vi "Assignment_Smart_Farming.vi"() -> ()   [LabVIEW 2020]
uses:
  <vilib>/MakerHub/LINX/Public/Peripherals/Digital/Digital Read 1 Chan.vi
  <vilib>/MakerHub/LINX/Public/Peripherals/Analog/Analog Read 1 Chan.vi
  <vilib>/MakerHub/LINX/Public/Peripherals/Digital/Digital Read N Chans.vi
  <vilib>/MakerHub/LINX/Public/Peripherals/Analog/Analog Read N Chans.vi
  <vilib>/MakerHub/LINX/Private/Local IO/LinxDigitalRead.vi
  <vilib>/MakerHub/LINX/Public/Utilities/Check Channel.vi
  <vilib>/MakerHub/LINX/Private/Local IO/LinxAnalogRead.vi
  <vilib>/MakerHub/LINX/Public/Utilities/Open Serial.vi
  <vilib>/MakerHub/LINX/Private/Utilties/Generate Error.vi
  <vilib>/httpClient/PUTBuffer.vi
  <vilib>/MakerHub/LINX/Public/Sensors/Motion/Servo/Servo Set Pulse Width One Channel.vi
  <vilib>/MakerHub/LINX/Public/Sensors/Motion/Servo/Servo Close One Channel.vi
  <vilib>/MakerHub/LINX/Public/Sensors/Motion/Servo/Servo Open One Channel.vi
  <vilib>/httpClient/LabVIEWHTTPClient.lvlib
  <vilib>/MakerHub/LINX/LMH-LINX.lvlib
  <vilib>/MakerHub/LINX/Public/Sensors/Motion/Servo/Servo.lvlib
panel:
  out "body":string
  out "PIR":bool
  out "Irrigation Level Received":dbl(slide) scale=0.0..10.0
  out "Rain Sensor":dbl(knob) scale=0.0..10.0
  out "Soil Moisture":dbl(slide) scale=0.0..50.0
  in  "STOP":bool
  out "Temp ^C":u8(knob) scale=0.0..50.0
  out "Humidity %":u8(knob) scale=0.0..100.0
  out "Device Name":string
  out "Data Sent":string
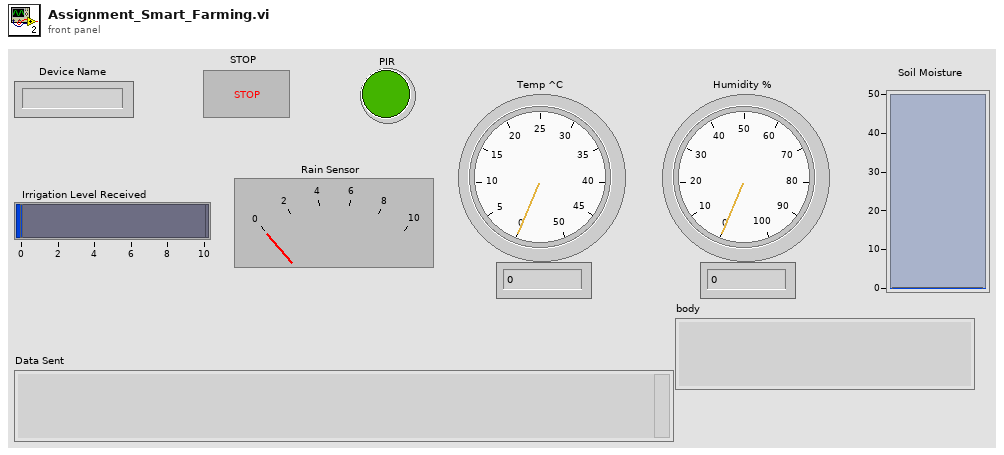
[diagram p1: front panel]
types:
  T1 = typedef "LMH-LINX.lvlib/LINX Ref.ctl" = cluster{"IO":T2, "Interface":T3, "LINX Device Config":T4}
  T2 = typedef "LMH-LINX.lvlib/Platform.ctl" = enum16{"Remote", "Local"}
  T3 = typedef "LMH-LINX.lvlib/Interface.ctl" = enum16{"Serial", "TCP"}
  T4 = typedef "LMH-LINX.lvlib/Device.lvlib/LINX Device Config.ctl" = cluster{"Interface":T3, "COM Port":refnum<visa-resource-name>, "TCP Configuration":T5, "Device Family":u8, "Device ID":u8, "Device Name":string, "TCP Ref":refnum<k5>, "Channels":T6}
  T5 = typedef "LMH-LINX.lvlib/Device.lvlib/TCP Config.ctl" = cluster{"IP Address":string, "Port":u16}
  T6 = typedef "LMH-LINX.lvlib/Channels.ctl" = cluster{"DI":u8[], "DO":u8[], "AI":u8[], "AO":u8[], "PWM":u8[], "QE":u8[], "UART":u8[], "I2C 2":u8[], "SPI":u8[], "CAN":u8[], "Servo":u8[], "AI Ref (V)":dbl, "AI Resolution (Bits)":u8, "AO Ref (V)":dbl, "AO Resolution (Bits)":u8}
  T7 = cluster{"Soil Moisture":dbl, "Rain":dbl, "Irrigation":string, "Humidity":i32, "Temperature":dbl, "PIR":bool}
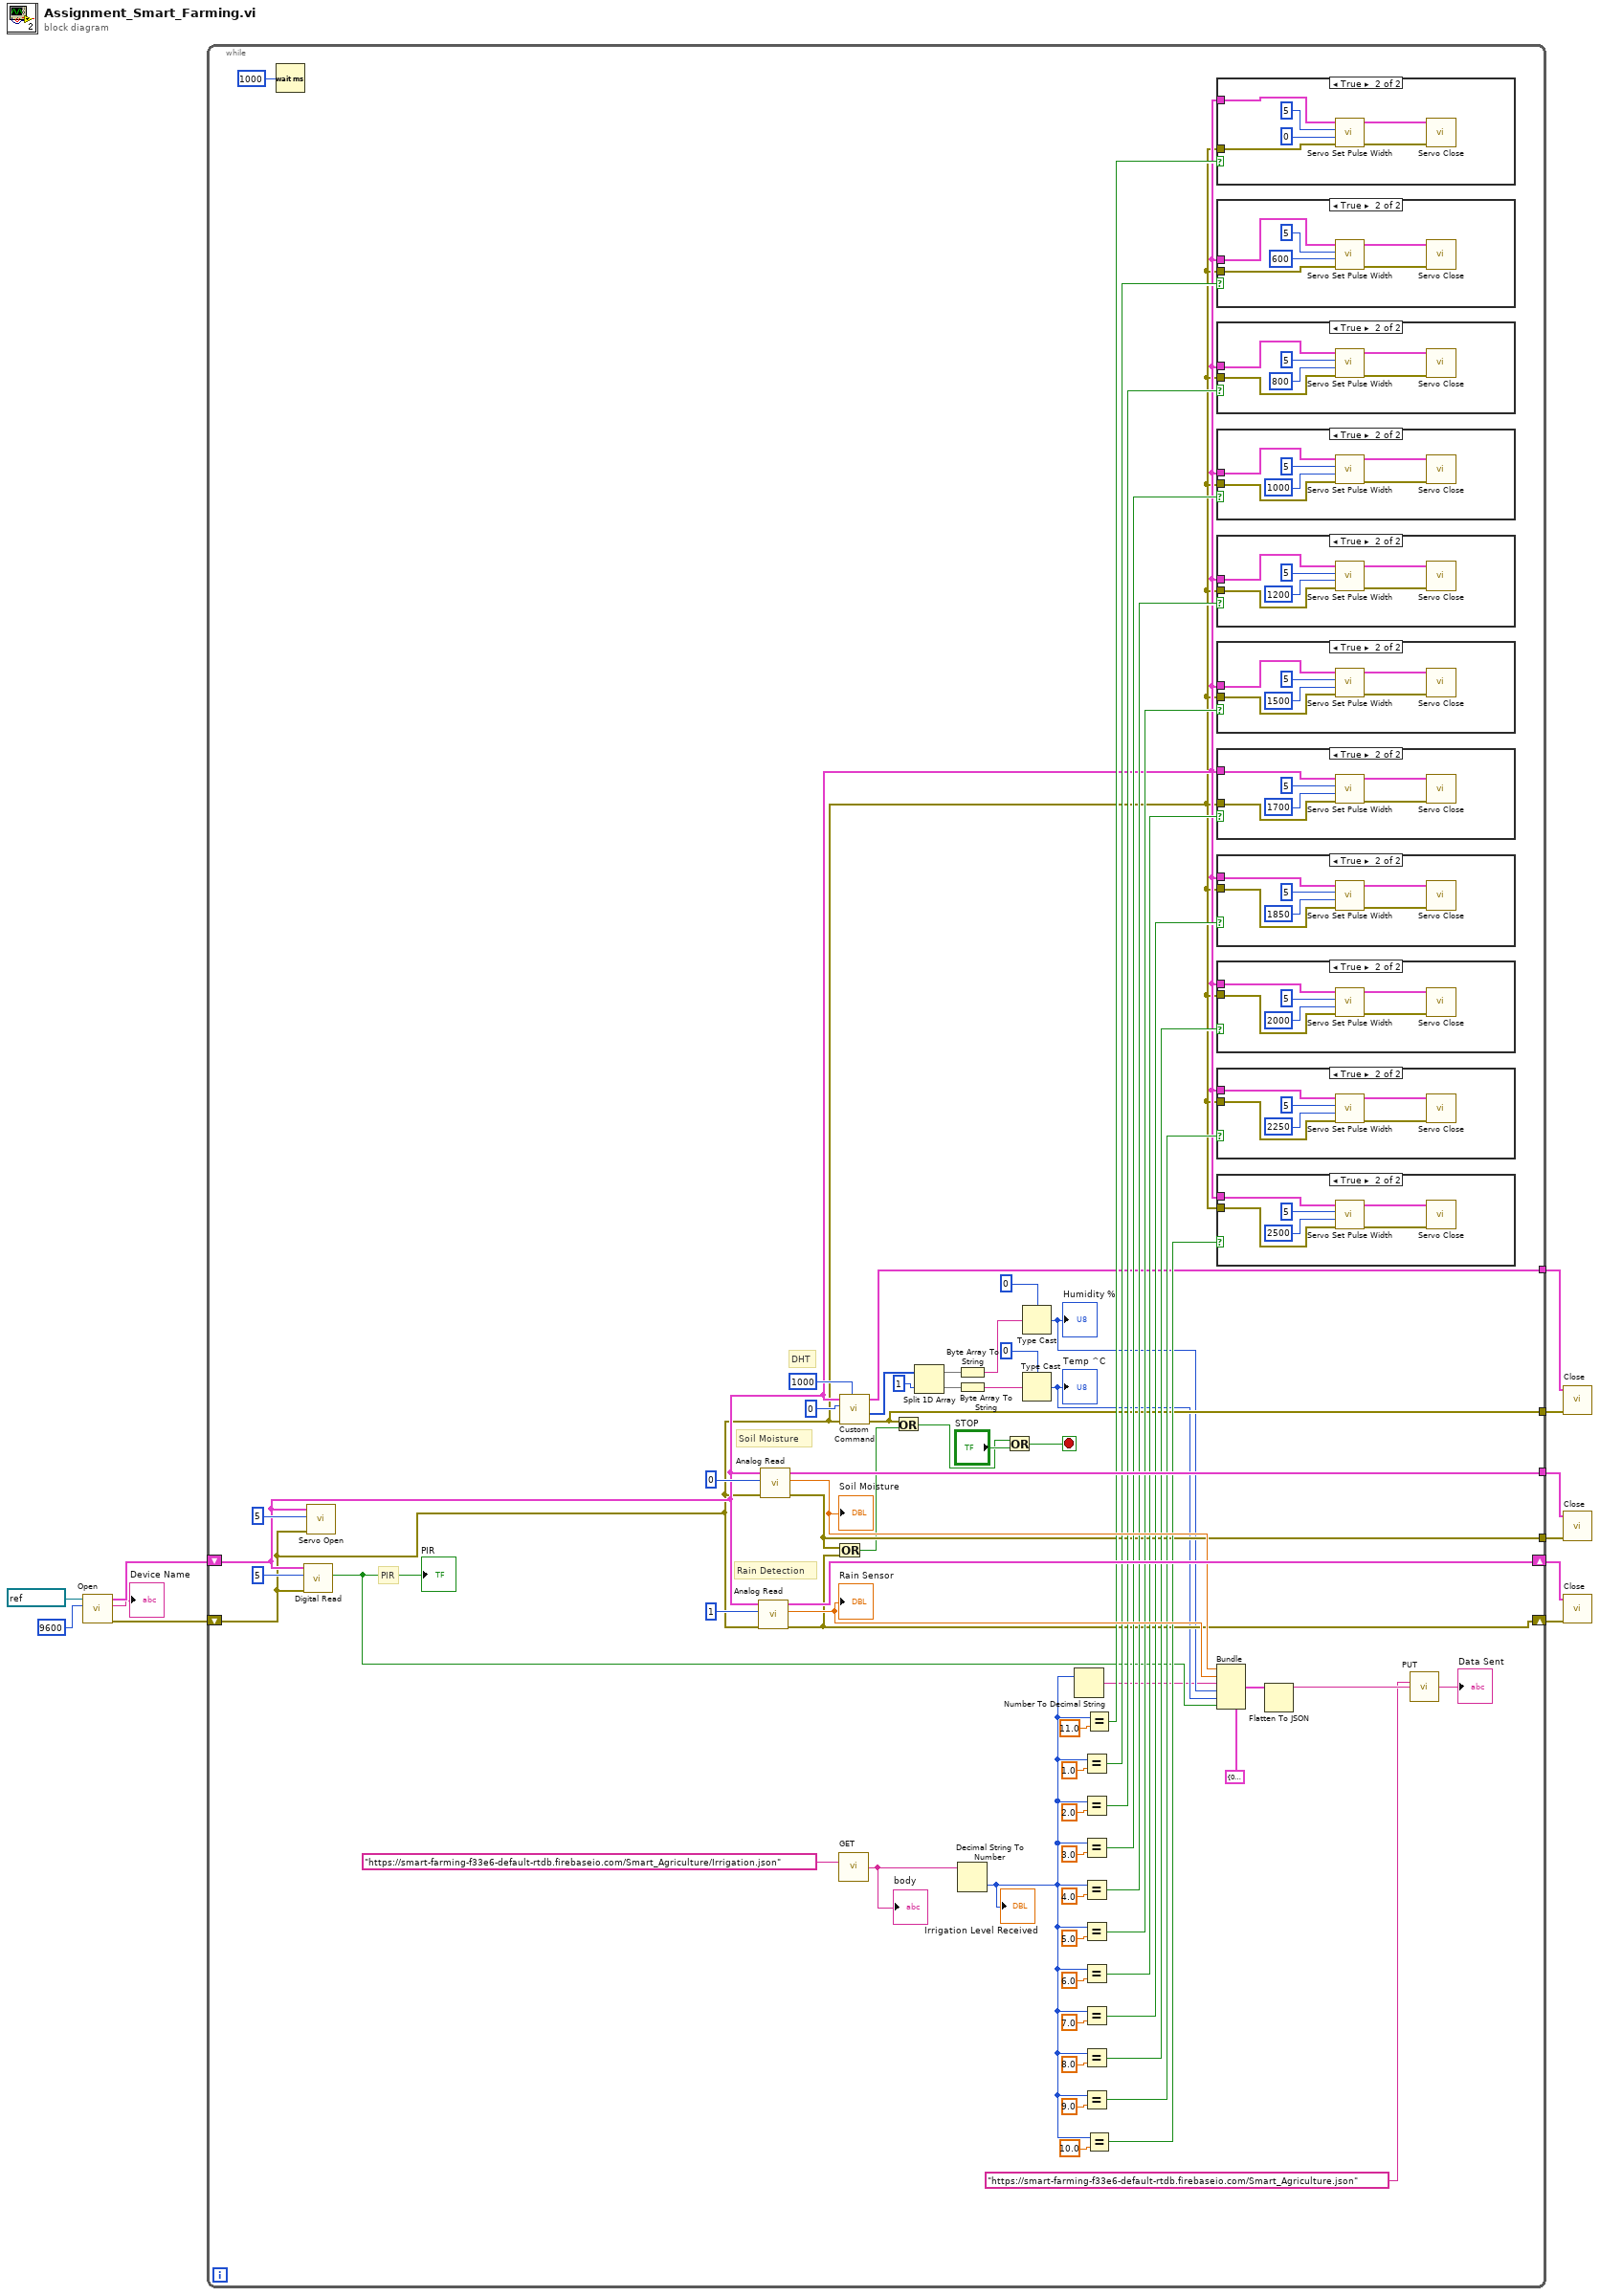
[diagram p0: block diagram]
diagram:
  n1 = call-poly <vilib>:"Open.vi"("Baud Rate Override"=u32 9600, "Serial Port"=refnum<visa-resource-name> "COM7") -> ("Error Out"=w8:errorcluster, "Device Name"=→"Device Name":string, "LINX Resource"=w9:T1)  [unwired: 7 in]
  n2 = while {
    tunnel: [w69] -> w5
    tunnel: [w28] -> w4
    shift-right: [w70] -> w7
    shift-left: w9 -> [w38]
    shift-right: [w27] -> w6
    shift-left: w8 -> [w37]
    tunnel: [w36] -> w2
    tunnel: [w26] -> w1
    stop <- w22 stop-if-true
    # "DHT"
    # "PIR"
    # "Rain Detection"
    # "Soil Moisture"
    n3 = Wait (ms)(milliseconds to wait=u32 1000) -> ()  [unwired: 1 out]
    n4 = call-poly <vilib>:"Digital Read.vi"("Error In"=w37, "DI Channel"=u8 5, "LINX Resource"=w38) -> ("DI Value"=w17:bool)  [unwired: 6 in, 2 out]
    "PIR" <- w17
    n5 = call-poly <vilib>:"Servo Open.vi"("Error In"=w37, "Servo Channel"=u8 5, "LINX Resource"=w38) -> ()  [unwired: 7 in, 2 out]
    n6 = call-poly <vilib>:"Analog Read.vi"("Error In"=w37, "Analog Channel"=u8 1, "LINX Resource"=w38) -> ("Error Out"=w27:errorcluster, "Voltage"=w64:dbl, "LINX Resource"=w70:T1)  [unwired: 5 in, 1 out]
    "Rain Sensor" <- w64
    n7 = call-poly <vilib>:"Analog Read.vi"("Error In"=w37, "Analog Channel"=u8 0, "LINX Resource"=w38) -> ("Error Out"=w28:errorcluster, "Voltage"=w65:dbl, "LINX Resource"=w69:T1)  [unwired: 5 in, 1 out]
    "Soil Moisture" <- w65
    n8 = Or(x=w28, y=w27) -> (x .or. y?=w25:bool)
    n9 = call <vilib>:"GET.vi"("url"="https://smart-farming-f33e6-default-rtdb.firebaseio.com/Smart_Agriculture/Irrigation.json") -> ("body"=w14:string)  [unwired: 11 in, 3 out]
    "body" <- w14
    n10 = call <vilib>:"Custom Command.vi"("Timeout (100 ms)"=1000, "Error In"=w37, "Custom Command Number"=u16 0, "LINX Resource"=w38) -> ("Error Out"=w26:errorcluster, "Response"=w20:u8[], "LINX Resource"=w36:T1)  [unwired: 4 in, 1 out]
    n11 = Or(x=w26, y=w25) -> (x .or. y?=w23:bool)
    n12 = Split 1D Array(array=w20, index=1) -> (first subarray=w34:u8[], second subarray=w33:u8[])
    n13 = Byte Array To String(unsigned byte array=w34) -> (string=w31:string)
    n14 = Byte Array To String(unsigned byte array=w33) -> (string=w29:string)
    n15 = Decimal String To Number(string=w14) -> (number=w13:i32)  [unwired: 2 in, 1 out]
    "Irrigation Level Received" <- w13
    n16 = Or(x=w23, y="STOP") -> (x .or. y?=w22:bool)
    n17 = Type Cast(type=u8 0, x=w31) -> (*(type *) &x=w19:u8)
    "Humidity %" <- w19
    n18 = Type Cast(type=u8 0, x=w29) -> (*(type *) &x=w21:u8)
    "Temp ^C" <- w21
    n19 = Number To Decimal String(number=w13) -> (decimal integer string=w12:string)  [unwired: 1 in]
    n20 = Equal?(x=w13, y=1.0) -> (x = y?=w59:bool)
    n21 = Equal?(x=w13, y=2.0) -> (x = y?=w57:bool)
    n22 = Equal?(x=w13, y=3.0) -> (x = y?=w55:bool)
    n23 = Equal?(x=w13, y=4.0) -> (x = y?=w53:bool)
    n24 = Equal?(x=w13, y=5.0) -> (x = y?=w51:bool)
    n25 = Equal?(x=w13, y=6.0) -> (x = y?=w49:bool)
    n26 = Equal?(x=w13, y=7.0) -> (x = y?=w47:bool)
    n27 = Equal?(x=w13, y=8.0) -> (x = y?=w45:bool)
    n28 = Equal?(x=w13, y=9.0) -> (x = y?=w43:bool)
    n29 = Equal?(x=w13, y=11.0) -> (x = y?=w62:bool)
    n30 = Equal?(x=w13, y=10.0) -> (x = y?=w41:bool)
    n31 = case shown="True" w62 {
      tunnel: w38 -> [_ w140]
      tunnel: w37 -> [_ w139]
      frame False {
      }
      frame True {
        n32 = call-poly <vilib>:"Servo Set Pulse Width.vi"("Error In"=w139, "Pulse Width (uS)"=u16 0, "Servo Channel"=u8 5, "LINX Resource"=w140) -> ("Error Out"=w135:errorcluster, "LINX Resource"=w136:T1)  [unwired: 6 in]
        n33 = call-poly <vilib>:"Servo Close.vi"("Error In"=w135, "LINX Resource"=w136) -> ()  [unwired: 8 in, 2 out]
      }
    }
    n34 = case shown="True" w59 {
      tunnel: w38 -> [_ w134]
      tunnel: w37 -> [_ w133]
      frame False {
      }
      frame True {
        n35 = call-poly <vilib>:"Servo Set Pulse Width.vi"("Error In"=w133, "Pulse Width (uS)"=u16 600, "Servo Channel"=u8 5, "LINX Resource"=w134) -> ("Error Out"=w129:errorcluster, "LINX Resource"=w130:T1)  [unwired: 6 in]
        n36 = call-poly <vilib>:"Servo Close.vi"("Error In"=w129, "LINX Resource"=w130) -> ()  [unwired: 8 in, 2 out]
      }
    }
    n37 = case shown="True" w57 {
      tunnel: w38 -> [_ w128]
      tunnel: w37 -> [_ w127]
      frame False {
      }
      frame True {
        n38 = call-poly <vilib>:"Servo Set Pulse Width.vi"("Error In"=w127, "Pulse Width (uS)"=u16 800, "Servo Channel"=u8 5, "LINX Resource"=w128) -> ("Error Out"=w123:errorcluster, "LINX Resource"=w124:T1)  [unwired: 6 in]
        n39 = call-poly <vilib>:"Servo Close.vi"("Error In"=w123, "LINX Resource"=w124) -> ()  [unwired: 8 in, 2 out]
      }
    }
    n40 = case shown="True" w55 {
      tunnel: w38 -> [_ w122]
      tunnel: w37 -> [_ w121]
      frame False {
      }
      frame True {
        n41 = call-poly <vilib>:"Servo Set Pulse Width.vi"("Error In"=w121, "Pulse Width (uS)"=u16 1000, "Servo Channel"=u8 5, "LINX Resource"=w122) -> ("Error Out"=w117:errorcluster, "LINX Resource"=w118:T1)  [unwired: 6 in]
        n42 = call-poly <vilib>:"Servo Close.vi"("Error In"=w117, "LINX Resource"=w118) -> ()  [unwired: 8 in, 2 out]
      }
    }
    n43 = case shown="True" w53 {
      tunnel: w38 -> [_ w116]
      tunnel: w37 -> [_ w115]
      frame False {
      }
      frame True {
        n44 = call-poly <vilib>:"Servo Set Pulse Width.vi"("Error In"=w115, "Pulse Width (uS)"=u16 1200, "Servo Channel"=u8 5, "LINX Resource"=w116) -> ("Error Out"=w111:errorcluster, "LINX Resource"=w112:T1)  [unwired: 6 in]
        n45 = call-poly <vilib>:"Servo Close.vi"("Error In"=w111, "LINX Resource"=w112) -> ()  [unwired: 8 in, 2 out]
      }
    }
    n46 = case shown="True" w51 {
      tunnel: w38 -> [_ w110]
      tunnel: w37 -> [_ w109]
      frame False {
      }
      frame True {
        n47 = call-poly <vilib>:"Servo Set Pulse Width.vi"("Error In"=w109, "Pulse Width (uS)"=u16 1500, "Servo Channel"=u8 5, "LINX Resource"=w110) -> ("Error Out"=w105:errorcluster, "LINX Resource"=w106:T1)  [unwired: 6 in]
        n48 = call-poly <vilib>:"Servo Close.vi"("Error In"=w105, "LINX Resource"=w106) -> ()  [unwired: 8 in, 2 out]
      }
    }
    n49 = case shown="True" w49 {
      tunnel: w38 -> [_ w104]
      tunnel: w37 -> [_ w103]
      frame False {
      }
      frame True {
        n50 = call-poly <vilib>:"Servo Set Pulse Width.vi"("Error In"=w103, "Pulse Width (uS)"=u16 1700, "Servo Channel"=u8 5, "LINX Resource"=w104) -> ("Error Out"=w99:errorcluster, "LINX Resource"=w100:T1)  [unwired: 6 in]
        n51 = call-poly <vilib>:"Servo Close.vi"("Error In"=w99, "LINX Resource"=w100) -> ()  [unwired: 8 in, 2 out]
      }
    }
    n52 = case shown="True" w47 {
      tunnel: w38 -> [_ w98]
      tunnel: w37 -> [_ w97]
      frame False {
      }
      frame True {
        n53 = call-poly <vilib>:"Servo Set Pulse Width.vi"("Error In"=w97, "Pulse Width (uS)"=u16 1850, "Servo Channel"=u8 5, "LINX Resource"=w98) -> ("Error Out"=w93:errorcluster, "LINX Resource"=w94:T1)  [unwired: 6 in]
        n54 = call-poly <vilib>:"Servo Close.vi"("Error In"=w93, "LINX Resource"=w94) -> ()  [unwired: 8 in, 2 out]
      }
    }
    n55 = case shown="True" w45 {
      tunnel: w38 -> [_ w92]
      tunnel: w37 -> [_ w91]
      frame False {
      }
      frame True {
        n56 = call-poly <vilib>:"Servo Set Pulse Width.vi"("Error In"=w91, "Pulse Width (uS)"=u16 2000, "Servo Channel"=u8 5, "LINX Resource"=w92) -> ("Error Out"=w87:errorcluster, "LINX Resource"=w88:T1)  [unwired: 6 in]
        n57 = call-poly <vilib>:"Servo Close.vi"("Error In"=w87, "LINX Resource"=w88) -> ()  [unwired: 8 in, 2 out]
      }
    }
    n58 = case shown="True" w43 {
      tunnel: w38 -> [_ w86]
      tunnel: w37 -> [_ w85]
      frame False {
      }
      frame True {
        n59 = call-poly <vilib>:"Servo Set Pulse Width.vi"("Error In"=w85, "Pulse Width (uS)"=u16 2250, "Servo Channel"=u8 5, "LINX Resource"=w86) -> ("Error Out"=w81:errorcluster, "LINX Resource"=w82:T1)  [unwired: 6 in]
        n60 = call-poly <vilib>:"Servo Close.vi"("Error In"=w81, "LINX Resource"=w82) -> ()  [unwired: 8 in, 2 out]
      }
    }
    n61 = case shown="True" w41 {
      tunnel: w38 -> [_ w80]
      tunnel: w37 -> [_ w79]
      frame False {
      }
      frame True {
        n62 = call-poly <vilib>:"Servo Set Pulse Width.vi"("Error In"=w79, "Pulse Width (uS)"=u16 2500, "Servo Channel"=u8 5, "LINX Resource"=w80) -> ("Error Out"=w75:errorcluster, "LINX Resource"=w76:T1)  [unwired: 6 in]
        n63 = call-poly <vilib>:"Servo Close.vi"("Error In"=w75, "LINX Resource"=w76) -> ()  [unwired: 8 in, 2 out]
      }
    }
    n64 = Bundle "Bundle"(cluster=T7 {"Soil Moisture"=0.0, "Rain"=1.0, "Irrigation"="", "Humidity"=4, "Temperature"=5.0, "PIR"=TRUE}, "Soil Moisture"=w65, "Rain"=w64, "Irrigation"=w12, "Humidity"=w19, "Temperature"=w21, "PIR"=w17) -> (w67:T7)
    n65 = Flatten To JSON(anything=w67) -> (JSON string=w74:string)  [unwired: 2 in, 1 out]
    n66 = call-poly <vilib>:"PUT.vi"("url"="https://smart-farming-f33e6-default-rtdb.firebaseio.com/Smart_Agriculture.json", "buffer"=w74) -> ("body"=→"Data Sent":string)  [unwired: 10 in, 3 out]
  }
  n67 = call <vilib>:"Close.vi"("Error In"=w1, "LINX Resource"=w2) -> ()  [unwired: 9 in, 1 out]
  n68 = call <vilib>:"Close.vi"("Error In"=w4, "LINX Resource"=w5) -> ()  [unwired: 9 in, 1 out]
  n69 = call <vilib>:"Close.vi"("Error In"=w6, "LINX Resource"=w7) -> ()  [unwired: 9 in, 1 out]
